vi "Check Address Match.vi"(8 "error in (no error)":errorcluster, 10 "Address":string, 11 "IP Resolver in":refnum<class "IP Resolver.lvclass">) -> (0 "error out":errorcluster, 2 "Matches":bool, 3 "IP Resolver out":refnum<class "IP Resolver.lvclass">)   [LabVIEW 2020, in "Vecto.lvlib" / "IP Resolver.lvclass"]
uses:
  IP Resolver.lvclass
  IP Resolver.lvclass/IP Resolver.ctl
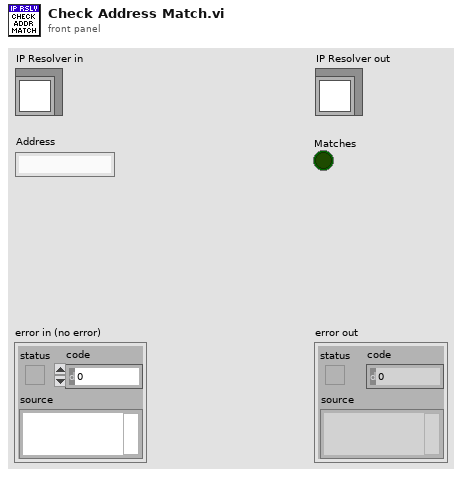
[diagram p1: front panel]
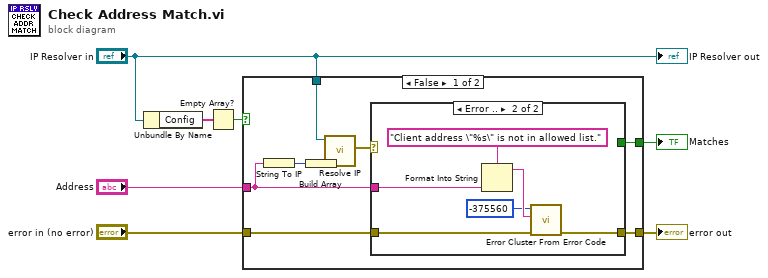
[diagram p0: block diagram]
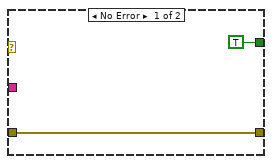
[diagram p2: hidden frame]
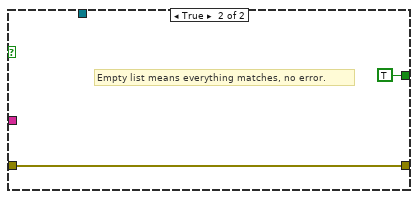
[diagram p3: hidden frame]
diagram:
  n1 = Unbundle By Name("IP Resolver in") -> ("Config"=w3:string[])
  n2 = Empty Array?(array=w3) -> (empty?=w2:bool)
  n3 = case shown="False" w2 {
    tunnel: "Address" -> [w12 _]
    tunnel: "error in (no error)" -> [w11 w25]
    tunnel: [w10 w25] -> w5
    tunnel: "IP Resolver in" -> [w9 _]
    tunnel: [w8 TRUE] -> w1
    frame False {
      n4 = String To IP(1:w12) -> (0:w15:u32)
      n5 = Build Array(w15) -> (w14:u32[])
      n6 = call "Resolve IP.vi"("Addresses (All)"=w14, "IP Resolver in"=w9) -> ("error out"=w13:errorcluster)  [unwired: 8 in, 1 out]
      n7 = case shown="Error .." w13 {
        tunnel: w12 -> [_ w23]
        tunnel: w11 -> [w17 w20]
        tunnel: [w17 w21] -> w10
        tunnel: [TRUE _] -> w8
        frame No Error {
        }
        frame Error {
          n8 = Format Into String(format string="Client address \"%s\" is not in allowed list.", w23) -> (resulting string=w19:string)  [unwired: 2 in, 1 out]
          n9 = call <vilib>:"Error Cluster From Error Code.vi"("error in (no error)"=w20, "error message (\"\")"=w19, "error code (0)"=-375560) -> ("error out"=w21:errorcluster)  [unwired: 6 in]
        }
      }
    }
    frame True {
      # "Empty list means everything matches, no error."
    }
  }
  "error out" <- w5
  "Matches" <- w1
  "IP Resolver out" <- "IP Resolver in"
